vi "initialise global varibales.vi"(8 "error in (no error)":errorcluster, 11 "focus in":refnum<class "focus.lvclass">) -> (0 "error out":errorcluster, 3 "focus out":refnum<class "focus.lvclass">)   [LabVIEW 2012, in "focus.lvclass"]
uses:
  focus.lvclass
  StageSPIM/PI drivers/Low Level/Communication.llb/Available interfaces.ctl
  StageSPIM/PI drivers/Low Level/Communication.llb/Available DLLs.ctl
  focus.lvclass/focus.ctl
  StageSPIM/PI drivers/Low Level/Communication.llb/Available DLL interfaces.ctl
  StageSPIM/PI drivers/Low Level/Communication.llb/Global1.vi
  StageSPIM/PI drivers/Low Level/Communication.llb/Global DaisyChain.vi
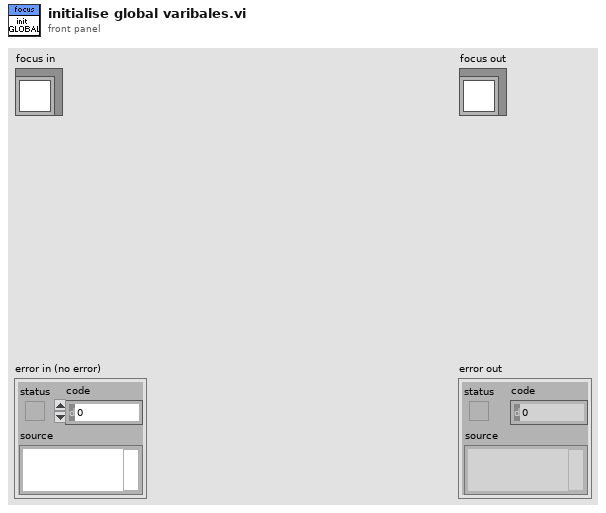
[diagram p1: front panel]
types:
  T1 = enum16{"C844_IsDLLAvailable", "C844_ConnectRS232", "C844_ConnectNIgpib", "C844_IsConnected", "C844_CloseConnection", "C844_GcsCommandset", "C844_GetError", "C844_GcsGetAnswerSize", "C844_GcsGetAnswer", "C843_IsDLLAvailable", "C843_Connect", "C843_IsConnected", "C843_CloseConnection", "C843_GcsCommandset", "C843_GetError", "C843_GcsGetAnswerSize", "C843_GcsGetAnswer", "E710_IsDLLAvailable", "E710_ConnectRS232", "E710_ConnectNIgpib", "E710_IsConnected", "E710_CloseConnection", "E710_GcsCommandset", "E710_GetError", "E710_GcsGetAnswerSize", "E710_GcsGetAnswer", "C843_PM_IsDLLAvailable", "C843_PM_Connect", "C843_PM_IsConnected", "C843_PM_CloseConnection", "C843_PM_GcsCommandset", "C843_PM_GetError", "C843_PM_GcsGetAnswerSize", "C843_PM_GcsGetAnswer", "C843_PM_GetCurrentBoardID", "C843_GetCurrentBoardID", "C865_IsDLLAvailable", "C865_ConnectRS232", "C865_IsConnected", "C865_CloseConnection", "C865_GcsCommandset", "C865_GetError", "C865_GcsGetAnswerSize", "C865_GcsGetAnswer", "C865_GetCurrentInterfaceID", "E761_ConnectPciBoard", "DefineSystem", "CloseConnection", "IsConnected", "ConnectRS232", "ConnectNIgpib", "ConnectPciBoard", "ConnectTCPIP", "GetError", "GcsCommandset", "GCSGetAnswerSize", "GcsGetAnswer"}
  T2 = enum16{"C844_IsDLLAvailable", "C844_ConnectRS232", "C844_ConnectNIgpib", "C844_IsConnected", "C844_CloseConnection", "C844_GcsCommandset", "C844_GetError", "C844_GcsGetAnswerSize", "C844_GcsGetAnswer", "C843_IsDLLAvailable", "C843_Connect", "C843_IsConnected", "C843_CloseConnection", "C843_GcsCommandset", "C843_GetError", "C843_GcsGetAnswerSize", "C843_GcsGetAnswer", "E710_IsDLLAvailable", "E710_ConnectRS232", "E710_ConnectNIgpib", "E710_IsConnected", "E710_CloseConnection", "E710_GcsCommandset", "E710_GetError", "E710_GcsGetAnswerSize", "E710_GcsGetAnswer", "C843_PM_IsDLLAvailable", "C843_PM_Connect", "C843_PM_IsConnected", "C843_PM_CloseConnection", "C843_PM_GcsCommandset", "C843_PM_GetError", "C843_PM_GcsGetAnswerSize", "C843_PM_GcsGetAnswer", "C843_PM_GetCurrentBoardID", "C843_GetCurrentBoardID", "C865_IsDLLAvailable", "C865_ConnectRS232", "C865_IsConnected", "C865_CloseConnection", "C865_GcsCommandset", "C865_GetError", "C865_GcsGetAnswerSize", "C865_GcsGetAnswer", "C865_GetCurrentInterfaceID", "E761_ConnectPciBoard", "DefineSystem", "CloseConnection", "IsConnected", "ConnectRS232", "ConnectNIgpib", "ConnectPciBoard", "ConnectTCPIP", "GetError", "GcsCommandset", "GCSGetAnswerSize", "GcsGetAnswer", "CloseDaisyChain", "OpenRS232DaisyChain", "ConnectDaisyChainDevice", "ConnectUSB", "ListUSB", "OpenUSBDaisyChain"}
  T3 = typedef "Available DLLs.ctl" = u16
  T4 = typedef "Available interfaces.ctl" = u16
  T5 = typedef "focus.lvclass/connection_type_focus.ctl" = enum16{"RS232", "RS232 DaisyChain", "USB", "USB_DaisyChain"}
  T6 = typedef "focus.lvclass/port_focus.ctl" = i32
  T7 = typedef "focus.lvclass/baud_rate_focus.ctl" = u16
  T8 = typedef "Available DLL interfaces.ctl" = u16
  T9 = cluster{"DLL for Device":T3, "DLL Interface":T8, "Parameter":string}[]
  T10 = cluster{"RS232 Portnumber":i32, "Timeout":i32, "RS232 Baud rate":u32, "Interface":T4, "GPIB Bus":i32, "GPIB Address":i32, "GPIB Mode":i32}[]
  T11 = cluster{"input XON/XOFF":bool, "input HW Handshake":bool, "input alt HW HShk":bool, "output XON/XOFF":bool, "output HW Handshake":bool, "output alt HW HShk":bool, "XOFF byte ":u8, "XON byte":u8, "parity error byte":u16}[]
  T12 = cluster{"input XON/XOFF":bool, "input HW Handshake":bool, "input alt HW HShk":bool, "output XON/XOFF":bool, "output HW Handshake":bool, "output alt HW HShk":bool, "XOFF byte ":u8, "XON byte":u8, "parity error byte":u16}
  T13 = cluster{"RS232 Portnumber":i32, "Timeout":i32, "RS232 Baud rate":u32, "Interface":T4, "GPIB Bus":i32, "GPIB Address":i32, "GPIB Mode":i32}
  T14 = cluster{"DLL for Device":T3, "DLL Interface":T8, "Parameter":string}
  T15 = cluster{"No. of devices":i32, "Port ID":i32, "Devices":string[], "Description":string}[]
  T16 = cluster{"No. of devices":i32, "Port ID":i32, "Devices":string[], "Description":string}
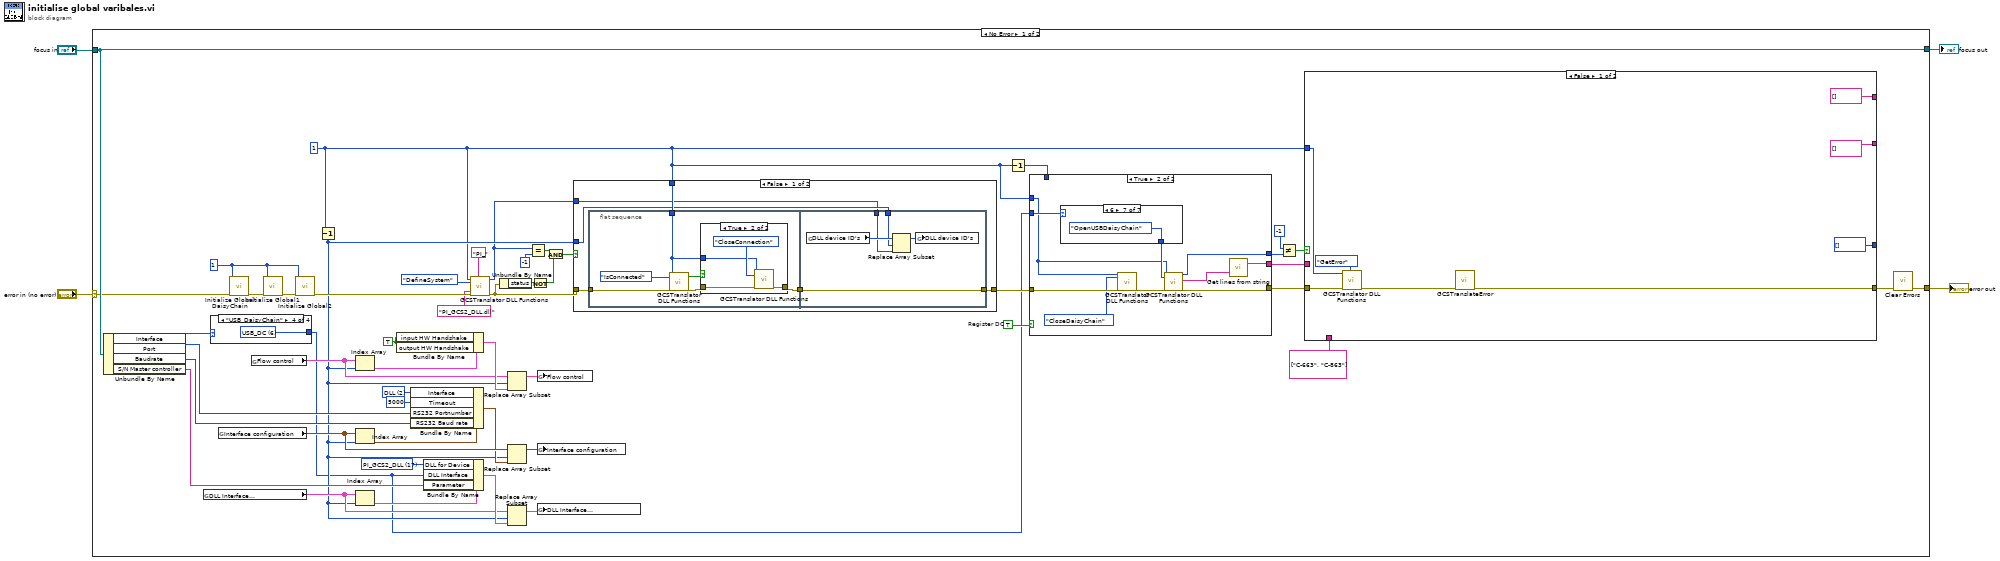
[diagram p0: block diagram]
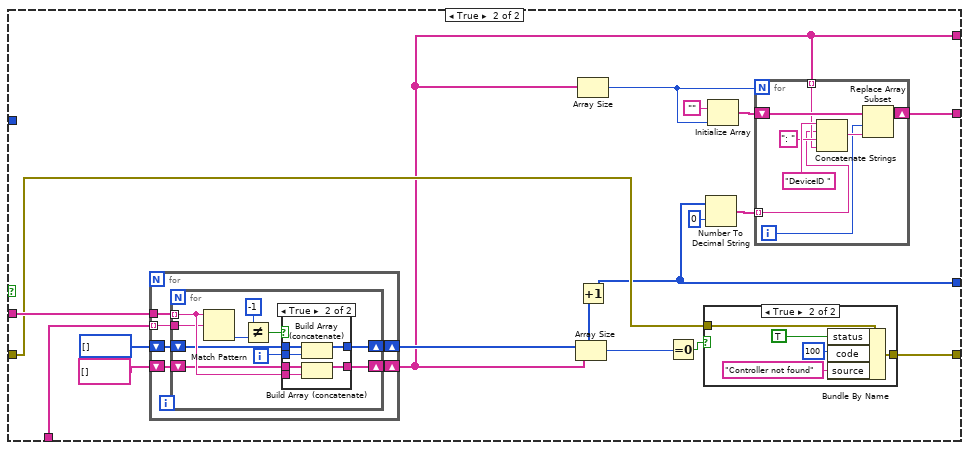
[diagram p2: hidden frame]
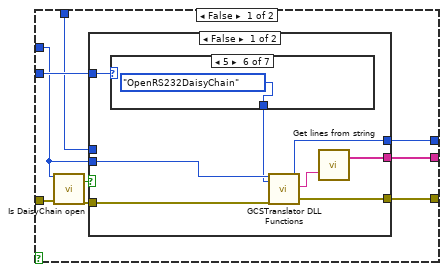
[diagram p5: hidden frame]
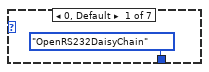
[diagram p6: hidden frame]
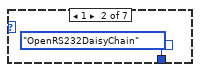
[diagram p7: hidden frame]
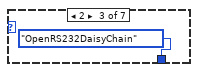
[diagram p8: hidden frame]
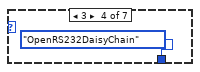
[diagram p9: hidden frame]
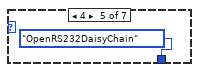
[diagram p10: hidden frame]
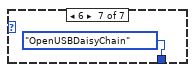
[diagram p11: hidden frame]
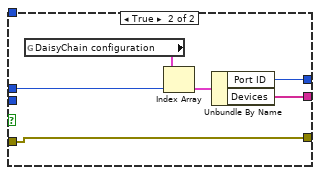
[diagram p12: hidden frame]
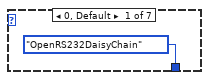
[diagram p13: hidden frame]
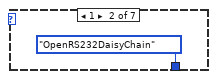
[diagram p14: hidden frame]
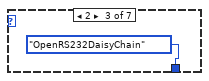
[diagram p15: hidden frame]
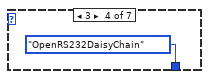
[diagram p16: hidden frame]
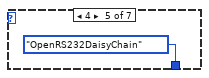
[diagram p17: hidden frame]
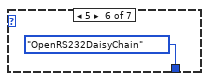
[diagram p18: hidden frame]
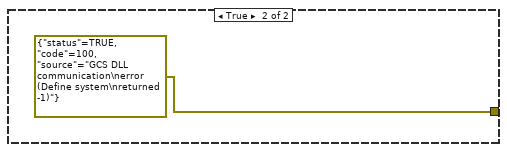
[diagram p20: hidden frame]
diagram:
  n1 = case shown="No Error" "error in (no error)" {
    selector: "error in (no error)" -> [w53 w193]
    tunnel: [w11 w193] -> w3
    tunnel: [w54 w192] -> w1
    tunnel: "focus in" -> [w54 w192]
    frame No Error {
      w17 = TRUE  # Register DC
      w25 = T3 17 items=["C-843", "C-844", "E-710", "C-843.PM", "C-865", "E-761", "Mercury", "E-755", "E-753", "C-866", "E-712", "E-725", "E-861", "C-867", "E-517", "E-816", "E-709", "PI_GCS2_DLL"] ("DLL for Device")
      w37 = T4 2 items=["RS232", "GPIB", "DLL", "TCP-IP", "USB", "Analog"] ("Interface")
      w6 = 1 ("System no.")
      w49 = TRUE ("Bundle Element")
      w50 = 1 ("System no.")
      n2 = Unbundle By Name(w54) -> ("Interface"=w35:T5, "Port"=w34:T6, "Baudrate"=w33:T7, "S/N Master controller"=w24:string)
      n3 = global read "Global1.vi" "DLL Interface\nConfiguration"() -> (w26:T9)
      n4 = case shown="\"USB_DaisyChain\"" w35 {
        tunnel: [w188 w189 w190 w191] -> w15
        frame "RS232", Default {
          w188 = T8 0 items=["RS232", "GPIB", "Board", "TCP-IP", "USB", "RS232_DC", "USB_DC"] ("DLL Interface")
        }
        frame "RS232 DaisyChain" {
          w189 = T8 5 items=["RS232", "GPIB", "Board", "TCP-IP", "USB", "RS232_DC", "USB_DC"] ("DLL Interface")
        }
        frame "USB" {
          w190 = T8 4 items=["RS232", "GPIB", "Board", "TCP-IP", "USB", "RS232_DC", "USB_DC"] ("DLL Interface")
        }
        frame "USB_DaisyChain" {
          w191 = T8 6 items=["RS232", "GPIB", "Board", "TCP-IP", "USB", "RS232_DC", "USB_DC"] ("DLL Interface")
        }
      }
      n5 = global read "Global1.vi" "Interface configuration"() -> (w32:T10)
      n6 = call "Initialize Global DaisyChain.vi"("System no."=w50, "error in"=w53) -> ("error out"=w52:errorcluster)  [unwired: 17 in]
      n7 = global read "Global1.vi" "Flow control"() -> (w20:T11)
      n8 = call "Initialize Global1.vi"("System no."=w50, "error in"=w52) -> ("error out"=w51:errorcluster)  [unwired: 17 in]
      n9 = call "Initialize Global2.vi"("System no."=w50, "error in"=w51) -> ("error out"=w48:errorcluster)  [unwired: 17 in]
      n10 = Decrement(x=w6) -> (x-1=w19:i32)
      n11 = Index Array(array=w20, index=w19) -> (element=w23:T12)
      n12 = Index Array(array=w32, index=w19) -> (element=w38:T13)
      n13 = Index Array(array=w26, index=w19) -> (element=w29:T14)
      n14 = Bundle By Name(cluster=w23, "input HW Handshake"=w49, "output HW Handshake"=w49) -> (w21:T12)
      n15 = Bundle By Name(cluster=w38, "Interface"=w37, "Timeout"=5000, "RS232 Portnumber"=w34, "RS232 Baud rate"=w33) -> (w31:T13)
      n16 = Bundle By Name(cluster=w29, "DLL for Device"=w25, "DLL Interface"=w15, "Parameter"=w24) -> (w27:T14)
      n17 = call "GCSTranslator DLL Functions.vi"("System no."=w6, "Function"=T1."DefineSystem", "String input"="PI_GCS2_DLL.dll", "error in"=w48, "String input 2"="PI_") -> ("DLL I32 Return value"=w18:i32, "error out"=w39:errorcluster)  [unwired: 10 in, 3 out]
      n18 = Unbundle By Name(w39) -> ("status"=w43:bool)
      n19 = Replace Array Subset(array=w20, new element=w21, index=w19) -> (w22:T11)
      n20 = Replace Array Subset(array=w32, new element=w31, index=w19) -> (w30:T10)
      n21 = Replace Array Subset(array=w26, new element=w27, index=w19) -> (w28:T9)
      n22 = Equal?(x=w18, y=-1) -> (x = y?=w42:bool)
      n23 = Not(x=w43) -> (.not. x?=w44:bool)
      n24 = global write "Global1.vi" "Flow control"(w22) -> ()
      n25 = global write "Global1.vi" "Interface configuration"(w30) -> ()
      n26 = global write "Global1.vi" "DLL Interface\nConfiguration"(w28) -> ()
      n27 = And(x=w42, y=w44) -> (x .and. y?=w40:bool)
      n28 = case shown="False" w40 {
        tunnel: w39 -> [w170 _]
        tunnel: w6 -> [w169 _]
        tunnel: [w167 errorcluster {"status"=TRUE, "code"=100, "source"="GCS DLL communication\nerror (Define system\nreturned -1)"} ("error out")] -> w16
        tunnel: w19 -> [w166 _]
        tunnel: w18 -> [w165 _]
        frame False {
          n29 = flat-sequence {
            tunnel: w170 -> [w175]
            tunnel: w169 -> [w172]
            tunnel: [w171] -> w168
            tunnel: w168 -> [w186]
            tunnel: [w186] -> w167
            tunnel: w166 -> [w183]
            tunnel: w165 -> [w182]
            frame #0 {
              n30 = call "GCSTranslator DLL Functions.vi"("System no."=w172, "Function"=T1."IsConnected", "error in"=w175) -> ("Boolean output"=w173:bool, "error out"=w174:errorcluster)  [unwired: 12 in, 3 out]
              n31 = case shown="True" w173 {
                tunnel: w174 -> [w177 w181]
                tunnel: w172 -> [_ w179]
                tunnel: [w177 w178] -> w171
                frame False {
                }
                frame True {
                  n32 = call "GCSTranslator DLL Functions.vi"("System no."=w179, "Function"=T1."CloseConnection", "error in"=w181) -> ("error out"=w178:errorcluster)  [unwired: 12 in, 4 out]
                }
              }
            }
            frame #1 {
              n33 = global read "Global1.vi" "DLL device ID's"() -> (w185:i32[])
              n34 = Replace Array Subset(array=w185, new element=w182, index=w183) -> (w184:i32[])
              n35 = global write "Global1.vi" "DLL device ID's"(w184) -> ()
            }
          }
        }
        frame True {
        }
      }
      n36 = Decrement(x=w6) -> (x-1=w14:i32)
      n37 = case shown="True" w17 {
        tunnel: w16 -> [w126 w156]
        tunnel: w15 -> [w123 w157]
        tunnel: w14 -> [w120 _]
        tunnel: [w122 w152] -> w8
        tunnel: w6 -> [w121 w151]
        tunnel: [w119 w150] -> w12
        tunnel: [w118 w149] -> w5
        frame False {
          n38 = call "Is DaisyChain open.vi"("System no."=w121, "error in"=w126) -> ("DC open?"=w124:bool, "error out"=w125:errorcluster)  [unwired: 15 in, 1 out]
          n39 = case shown="False" w124 {
            tunnel: w125 -> [w133 w147]
            tunnel: w123 -> [w134 _]
            tunnel: [w132 w147] -> w122
            tunnel: w121 -> [w131 _]
            tunnel: w120 -> [_ w146]
            tunnel: [w129 w143] -> w119
            tunnel: [w127 w142] -> w118
            frame False {
              n40 = case shown="5" w134 {
                tunnel: [T2."OpenRS232DaisyChain" ("Function") T2."OpenRS232DaisyChain" ("Function") T2."OpenRS232DaisyChain" ("Function") T2."OpenRS232DaisyChain" ("Function") T2."OpenRS232DaisyChain" ("Function") T2."OpenRS232DaisyChain" ("Function") T2."OpenUSBDaisyChain" ("Function")] -> w130
                frame 0, Default {
                }
                frame 1 {
                }
                frame 2 {
                }
                frame 3 {
                }
                frame 4 {
                }
                frame 5 {
                }
                frame 6 {
                }
              }
              n41 = call "GCSTranslator DLL Functions.vi"("System no."=w131, "Function"=w130, "error in"=w133) -> ("DLL I32 Return value"=w129:i32, "String output"=w128:string, "error out"=w132:errorcluster)  [unwired: 12 in, 2 out]
              n42 = call "Get lines from string.vi"("Input string"=w128) -> ("Strings"=w127:string[])  [unwired: 17 in, 1 out]
            }
            frame True {
              n43 = global read "Global DaisyChain.vi" "DaisyChain configuration"() -> (w145:T15)
              n44 = Index Array(array=w145, index=w146) -> (element=w144:T16)
              n45 = Unbundle By Name(w144) -> ("Port ID"=w143:i32, "Devices"=w142:string[])
            }
          }
        }
        frame True {
          n46 = case shown="6" w157 {
            tunnel: [T2."OpenRS232DaisyChain" ("Function") T2."OpenRS232DaisyChain" ("Function") T2."OpenRS232DaisyChain" ("Function") T2."OpenRS232DaisyChain" ("Function") T2."OpenRS232DaisyChain" ("Function") T2."OpenRS232DaisyChain" ("Function") T2."OpenUSBDaisyChain" ("Function")] -> w153
            frame 0, Default {
            }
            frame 1 {
            }
            frame 2 {
            }
            frame 3 {
            }
            frame 4 {
            }
            frame 5 {
            }
            frame 6 {
            }
          }
          n47 = call "GCSTranslator DLL Functions.vi"("System no."=w151, "Function"=T2."CloseDaisyChain", "error in"=w156) -> ("error out"=w155:errorcluster)  [unwired: 12 in, 4 out]
          n48 = call "GCSTranslator DLL Functions.vi"("System no."=w151, "Function"=w153, "error in"=w155) -> ("DLL I32 Return value"=w150:i32, "String output"=w148:string, "error out"=w152:errorcluster)  [unwired: 12 in, 2 out]
          n49 = call "Get lines from string.vi"("Input string"=w148) -> ("Strings"=w149:string[])  [unwired: 17 in, 1 out]
        }
      }
      n50 = Not Equal?(x=-1 ("y"), y=w12) -> (x != y?=w10:bool)
      n51 = case shown="False" w10 {
        tunnel: string[] ["C-663", "C-863"] -> [_ w69]
        tunnel: w8 -> [w61 w67]
        tunnel: [w55 w66] -> w7
        tunnel: w6 -> [w60 _]
        tunnel: [string[] [] w63] -> _
        tunnel: [string[] [] w64] -> _
        tunnel: [i32[] [] w65] -> _
        tunnel: w5 -> [_ w68]
        frame False {
          n52 = call "GCSTranslator DLL Functions.vi"("System no."=w60, "Function"=T2."GetError", "error in"=w61) -> ("error out"=w56:errorcluster)  [unwired: 12 in, 4 out]
          n53 = call "GCSTranslateError.vi"("error in"=w56) -> ("error out"=w55:errorcluster)  [unwired: 16 in, 2 out]
        }
        frame True {
          n54 = for {
            tunnel: w69 -> [w84] mode=indexing
            tunnel: w68 -> [w82]
            shift-right: [w83] -> w63
            shift-left: string[] [] -> [w85]
            shift-right: [w80] -> w70
            shift-left: i32[] [] -> [w81]
            n55 = for {
              tunnel: w82 -> [w93] mode=indexing
              shift-right: [w92] -> w83
              shift-left: w85 -> [w91]
              tunnel: w84 -> [w90]
              shift-right: [w89] -> w80
              shift-left: w81 -> [w88]
              i -> [w86]
              n56 = Match Pattern(string=w93, regular expression=w90) -> (offset past match=w87:i32)  [unwired: 1 in, 3 out]
              n57 = Not Equal?(x=-1 ("y"), y=w87) -> (x != y?=w94:bool)
              n58 = case shown="True" w94 {
                tunnel: w93 -> [_ w102]
                tunnel: [w97 w103] -> w92
                tunnel: w91 -> [w97 w101]
                tunnel: [w96 w100] -> w89
                tunnel: w88 -> [w96 w99]
                tunnel: w86 -> [_ w98]
                frame False {
                }
                frame True {
                  n59 = Build Array (concatenate)(w99, w98) -> (w100:i32[])
                  n60 = Build Array (concatenate)(w101, w102) -> (w103:string[])
                }
              }
            }
          }
          n61 = Array Size(array=w63) -> (size(s)=w75:i32)
          n62 = Array Size(array=w63) -> (size(s)=w77:i32)
          n63 = Increment(x=w70) -> (x+1=w65:i32[])
          n64 = Equal To 0?(x=w75) -> (x = 0?=w74:bool)
          n65 = case shown="True" w74 {
            tunnel: [w104 w106] -> w66
            tunnel: w67 -> [w104 w105]
            frame False {
            }
            frame True {
              n66 = Bundle By Name(cluster=w105, "status"=TRUE, "code"=100 ("Bundle Element"), "source"="Controller not found" ("Bundle Element")) -> (w106:errorcluster)
            }
          }
          n67 = Number To Decimal String(number=w65, width (-)=i16 0) -> (decimal integer string=w71:string[])
          n68 = Initialize Array("", w77) -> (w79:string[])
          n69 = for {
            N: w77 -> [_]
            shift-right: [w115] -> w64
            shift-left: w79 -> [w117]
            tunnel: w63 -> [w111] mode=indexing
            tunnel: w71 -> [w110] mode=indexing
            i -> [w113]
            n70 = Concatenate Strings("DeviceID ", w110, ": " ("string"), w111) -> (w116:string)
            n71 = Replace Array Subset(array=w117, new element=w116, index=w113) -> (w115:string[])
          }
        }
      }
      n72 = call <vilib>:"Clear Errors.vi"("error in (no error)"=w7) -> ("error out"=w11:errorcluster)  [unwired: 6 in]
    }
    frame Error {
    }
  }
  "error out" <- w3
  "focus out" <- w1
